vi "CIMAQ Overlay Rectangle Big.vi"(6 "Overlay Thickness":i32(slide)=5 scale=0.0..20.0, 7 "Color":u32(colorbox)=16711680, 8 "error in (no error)":errorcluster, 10 "Rectangle":T1, 11 "Image In":T2) -> (0 "error out":errorcluster, 3 "Image Out":T2)   [LabVIEW 2014]
uses:
  <vilib>/vision/Image Controls.llb/IMAQ Image.ctl
panel:
  in  "OverlayName":string
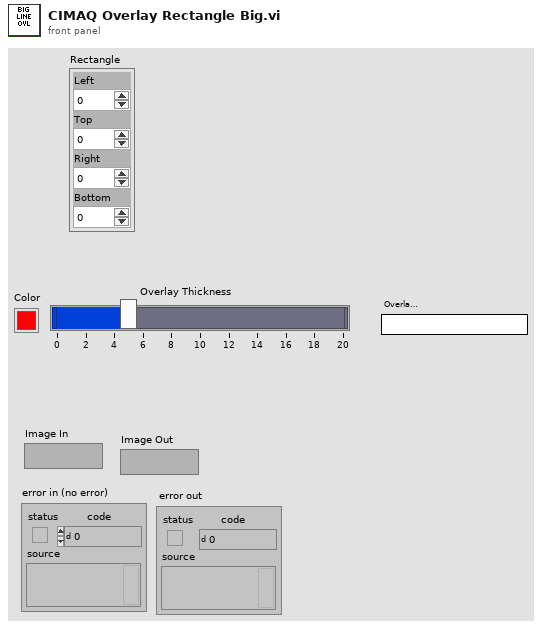
[diagram p1: front panel]
types:
  T1 = cluster{"Left":i32, "Top":i32, "Right":i32, "Bottom":i32}
  T2 = typedef "IMAQ Image.ctl" = refnum<image>
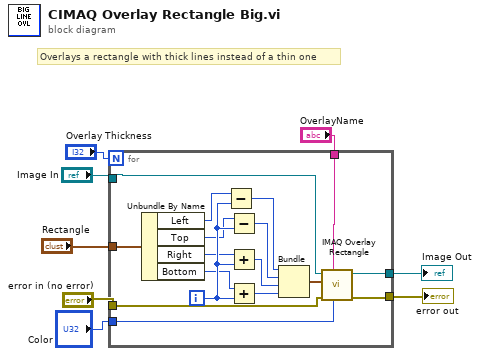
[diagram p0: block diagram]
diagram:
  # "Overlays a rectangle with thick lines instead of a thin one"
  n1 = for {
    N: "Overlay Thickness" -> [_]
    tunnel: "Image In" -> [w25]
    tunnel: "error in (no error)" -> [w24]
    tunnel: [w23] -> w3
    tunnel: "Rectangle" -> [w22]
    tunnel: "Color" -> [w11]
    tunnel: [w10] -> w2
    tunnel: "OverlayName" -> [w9]
    i -> [w21]
    n2 = Unbundle By Name(w22) -> ("Left"=w20:i32, "Top"=w19:i32, "Right"=w17:i32, "Bottom"=w18:i32)
    n3 = Subtract(x=w20, y=w21) -> (x-y=w16:i32)
    n4 = Subtract(x=w19, y=w21) -> (x-y=w15:i32)
    n5 = Add(x=w17, y=w21) -> (x+y=w14:i32)
    n6 = Add(x=w18, y=w21) -> (x+y=w13:i32)
    n7 = Bundle(w16, w15, w14, w13) -> (w12:cluster{i32, i32, i32, i32})  [unwired: 1 in]
    n8 = call "IMAQ Overlay Rectangle"("Color"=w11, "Group"=w9, "error in (no error)"=w24, "Rectangle"=w12, "Image"=w25) -> ("error out"=w10:errorcluster, "Image Out"=w23:T2)  [unwired: 5 in]
  }
  "Image Out" <- w3
  "error out" <- w2
